vi "Caldeck_Alicat_MFC.vi"() -> ()   [LabVIEW 2014]
uses:
  <vilib>/Instr/_visa.llb/VISA Configure Serial Port (Instr).vi
panel:
  out "status":bool
  out "Value Read":string
  in  "SLPM Value to be set":dbl=1.5
  in  "SET Value":bool
  in  "timeout (10sec)":u32=3000
  in  "VISA resource name":refnum<visa-resource-name>="ASRL13::INSTR"
  out "error out":errorcluster
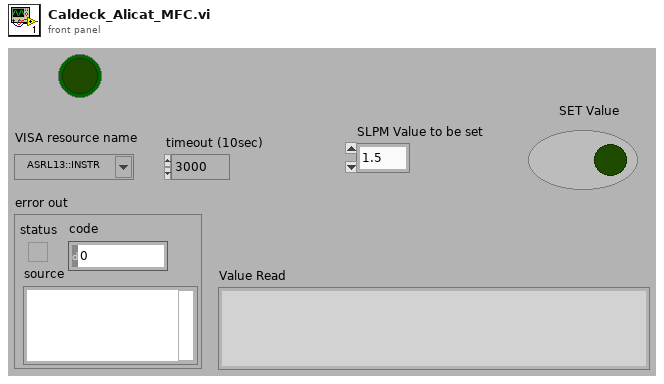
[diagram p1: front panel]
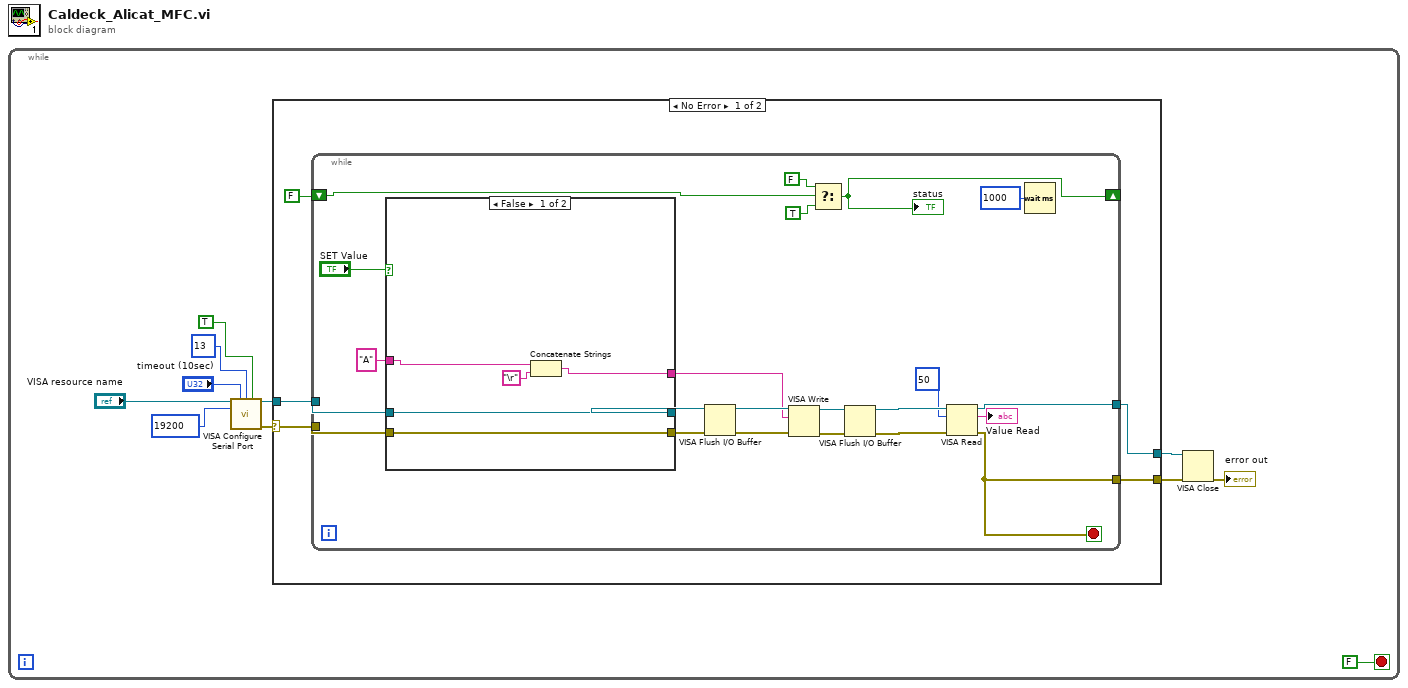
[diagram p0: block diagram]
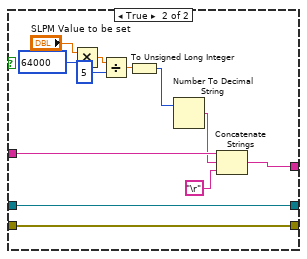
[diagram p2: hidden frame]
diagram:
  n1 = while {
    stop <- FALSE stop-if-true
    n2 = call-poly "VISA Configure Serial Port"("VISA resource name"="VISA resource name", "timeout (10sec)"="timeout (10sec)", "termination char\n(0xA = '\\n' = LF)"=u8 13 ("termination char\n(0xA = '\\n' = LF)"), "Enable Termination\nChar (T)"=TRUE ("Enable Termination\nChar (T)"), "baud rate (9600)"=u32 19200) -> ("VISA resource name out"=w11:refnum<visa-resource-name>, "error out"=w7:errorcluster)  [unwired: 9 in]
    n3 = case shown="No Error" w7 {
      selector: w7 -> [w15 w56]
      tunnel: w11 -> [w16 w57]
      tunnel: [w14 w57] -> w10
      tunnel: [w13 w56] -> w9
      frame No Error {
        n4 = while {
          tunnel: w16 -> [w34]
          tunnel: w15 -> [w32]
          tunnel: [w23] -> w14
          tunnel: [w17] -> w13
          shift-right: [w18] -> _
          shift-left: FALSE -> [w21]
          stop <- w17 stop-if-true
          n5 = case shown="False" "SET Value" {
            tunnel: w34 -> [w40 w55]
            tunnel: [w40 w55] -> w33
            tunnel: w32 -> [w39 w54]
            tunnel: [w39 w54] -> w31
            tunnel: "A" -> [w43 w47]
            tunnel: [w41 w44] -> w29
            frame False {
              n6 = Concatenate Strings(w43, "\r") -> (w41:string)
            }
            frame True {
              n7 = Multiply(x="SLPM Value to be set", y=u32 64000) -> (x*y=w51:dbl)
              n8 = Divide(x=w51, y=u32 5) -> (x/y=w49:dbl)
              n9 = To Unsigned Long Integer(number=w49) -> (unsigned 32bit integer=w48:u32)
              n10 = Number To Decimal String(number=w48) -> (decimal integer string=w46:string)  [unwired: 1 in]
              n11 = Concatenate Strings(w47, w46, "\r") -> (w44:string)
            }
          }
          n12 = VISA Flush I/O Buffer(VISA resource name=w33, error in (no error)=w31) -> (VISA resource name out=w36:refnum<visa-resource-name>, error out=w35:errorcluster)  [unwired: 1 in]
          n13 = VISA Write(VISA resource name=w36, write buffer=w29, error in (no error)=w35) -> (VISA resource name out=w28:refnum<visa-resource-name>, error out=w27:errorcluster)  [unwired: 1 out]
          n14 = Select(t=FALSE, s=w21, f=TRUE) -> (s? t:f=w18:bool)
          "status" <- w18
          n15 = VISA Flush I/O Buffer(VISA resource name=w28, error in (no error)=w27) -> (VISA resource name out=w38:refnum<visa-resource-name>, error out=w37:errorcluster)  [unwired: 1 in]
          n16 = VISA Read(VISA resource name=w38, byte count=u32 50, error in (no error)=w37) -> (VISA resource name out=w23:refnum<visa-resource-name>, read buffer=→"Value Read":string, error out=w17:errorcluster)  [unwired: 1 out]
          n17 = Wait (ms)(milliseconds to wait=u32 1000) -> ()  [unwired: 1 out]
        }
      }
      frame Error {
      }
    }
    n18 = VISA Close(VISA resource name=w10, error in (no error)=w9) -> (error out=→"error out":errorcluster)
  }
